vi "ATS_TimeStamp.vi"(10 "TimeStampLow":u32, 11 "TimeStampHigh":u32) -> (3 "TimeStamp_Clk":dbl)   [LabVIEW 2022 SP3]
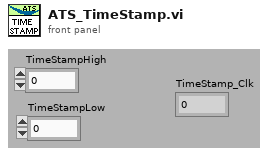
[diagram p1: front panel]
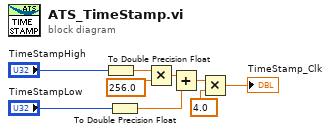
[diagram p0: block diagram]
diagram:
  n1 = To Double Precision Float(number="TimeStampHigh") -> (double precision float=w3:dbl)
  n2 = To Double Precision Float(number="TimeStampLow") -> (double precision float=w6:dbl)
  n3 = Multiply(x=w3, y=256.0) -> (x*y=w1:dbl)
  n4 = Add(x=w1, y=w6) -> (x+y=w5:dbl)
  n5 = Multiply(x=w5, y=4.0) -> (x*y=→"TimeStamp_Clk":dbl)
